vi "RunModelList.vi"(7 "Models":T1(c390), 11 "ModelList":refnum<vi>) -> ()   [LabVIEW 2025, in "Test Unit.lvlib"]
uses:
  Test Unit.lvlib
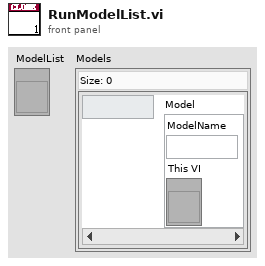
[diagram p1: front panel]
types:
  T1 = map{string, cluster{"ModelName":string, "This VI":refnum<vi>}}
  T2 = cluster{"Left Cell String":string, "Child Text":string[], "Child Tag":string, "Item Indent":i32, "Child Only?":bool, "Glyph Index":i32}
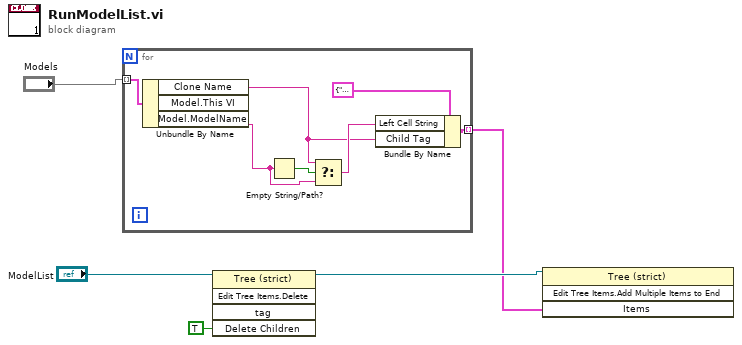
[diagram p0: block diagram]
diagram:
  n1 = for {
    tunnel: "Models" -> [w12] mode=indexing
    tunnel: [w6] -> w1 mode=indexing
    n2 = Unbundle By Name(w12) -> ("Clone Name"=w7:string, "Model.ModelName"=w9:string)  [unwired: 1 out]
    n3 = Empty String/Path?(string/path=w9) -> (empty?=w10:bool)
    n4 = Select(t=w7, s=w10, f=w9) -> (s? t:f=w8:string)
    n5 = Bundle By Name(cluster=T2 {"Left Cell String"="", "Child Text"=[], "Child Tag"="", "Item Indent"=0, "Child Only?"=FALSE, "Glyph Index"=0} ("Item"), "Left Cell String"=w8, "Child Tag"=w7) -> (w6:T2)
  }
  n6 = invoke class="Tree (strict)" method="Edit Tree Items.Delete"(reference="ModelList", "Delete Children"=TRUE ("Delete Children?")) -> (reference out=w3:refnum<vi>)  [unwired: 3 in, 4 out]
  n7 = invoke class="Tree (strict)" method="Edit Tree Items.Add Multiple Items to End"(reference=w3, "Items"=w1) -> ()  [unwired: 2 in, 4 out]
